vi "Read ref.vi"(8 "error in (no error)":errorcluster, 11 "DynamicParameters in":refnum<class "DapperParameters.lvclass">) -> (0 "error out":errorcluster, 2 "ref":T1, 3 "DynamicParameters out":refnum<class "DapperParameters.lvclass">)   [LabVIEW 2020, in "ORM_Dapper.lvlib" / "DapperParameters.lvclass"]
uses:
  DapperParameters.lvclass
  dapper_dynamicparameters_ref.ctl
  C:/Viviota/Projects/R&D/LabVIEW_ORM/source/src/libraries/dapper/Dapper.dll
  libraries/dapper/Dapper.dll
  DapperParameters.lvclass/DapperParameters.ctl
  ORM_Dapper.lvlib
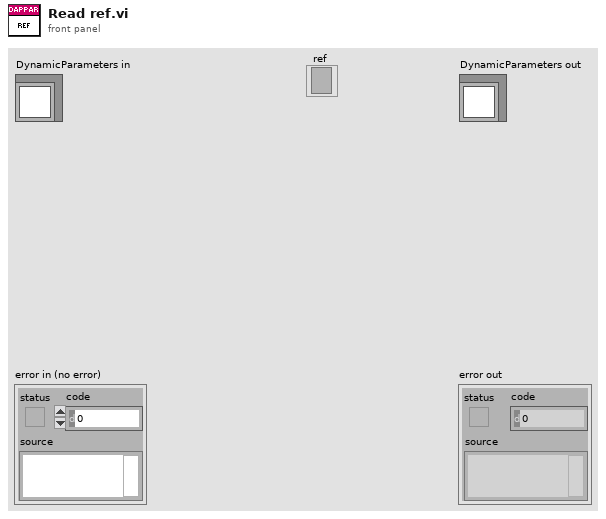
[diagram p1: front panel]
types:
  T1 = typedef "ORM_Dapper.lvlib/dapper_dynamicparameters_ref.ctl" = refnum<k24>
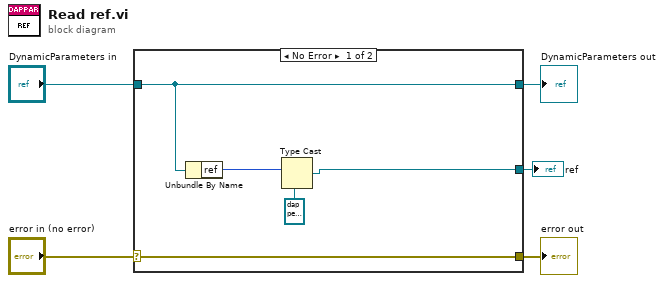
[diagram p0: block diagram]
diagram:
  n1 = case shown="No Error" "error in (no error)" {
    selector: "error in (no error)" -> [w9 w11]
    tunnel: [w9 w11] -> w4
    tunnel: [w10 w12] -> w2
    tunnel: "DynamicParameters in" -> [w10 w12]
    tunnel: [w7 _] -> w1
    frame No Error {
      n2 = Unbundle By Name(w10) -> ("ref"=w8:u64)
      n3 = Type Cast(type=T1 refnum ("ref"), x=w8) -> (*(type *) &x=w7:T1)
    }
    frame Error {
    }
  }
  "error out" <- w4
  "DynamicParameters out" <- w2
  "ref" <- w1
